vi "Delete All Case Structure Frames But Default.vi"(8 "error in (no error)":errorcluster, 11 "CaseStructure in":refnum<vi>) -> (0 "error out":errorcluster, 3 "CaseStructure out":refnum<vi>)   [LabVIEW 2019, in "gRPC Template Creation Utility.lvlib"]
uses:
  gRPC Template Creation Utility.lvlib
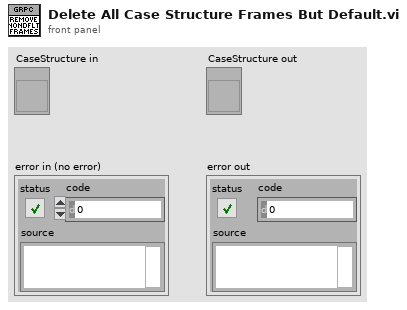
[diagram p1: front panel]
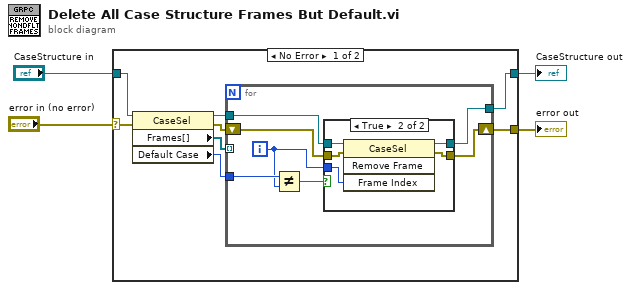
[diagram p0: block diagram]
diagram:
  n1 = case shown="No Error" "error in (no error)" {
    selector: "error in (no error)" -> [w7 w28]
    tunnel: [w10 w27] -> w4
    tunnel: [w5 w28] -> w3
    tunnel: "CaseStructure in" -> [w12 w27]
    frame No Error {
      n2 = property class="CaseSel"(reference=w12, error in=w7) -> (reference out=w8:refnum<vi>, error out=w6:errorcluster, "Frames[]"=w11:refnum<vi>[], "Default Case"=w9:i32)
      n3 = for {
        tunnel: w11 -> [_] mode=indexing
        tunnel: [w19] -> w10
        tunnel: w9 -> [w18]
        tunnel: w8 -> [w16]
        shift-right: [w13] -> w5
        shift-left: w6 -> [w14]
        i -> [w15]
        n4 = Not Equal?(x=w18, y=w15) -> (x != y?=w17:bool)
        n5 = case shown="True" w17 {
          tunnel: [w21 w26] -> w19
          tunnel: w16 -> [w21 w25]
          tunnel: w15 -> [_ w24]
          tunnel: w14 -> [w20 w23]
          tunnel: [w20 w22] -> w13
          frame False {
          }
          frame True {
            n6 = invoke class="CaseSel" method="Remove Frame"(reference=w25, error in=w23, "Frame Index"=w24) -> (reference out=w26:refnum<vi>, error out=w22:errorcluster)  [unwired: 1 in, 2 out]
          }
        }
      }
    }
    frame Error {
    }
  }
  "error out" <- w3
  "CaseStructure out" <- w4
